vi "Plot PSD.vi"(6 "averaging parameters":T1={"averaging mode"=enum."No averaging", "weighting mode"=enum."Exponential", "number of averages"=10} {"number of averages" min=1}, 7 "restart averaging (F)":bool, 8 "error in (no error)":errorcluster, 9 "dB On (F)":bool, 10 "window":T2=1 items=["Rectangle"=0, "Hanning"=1, "Hamming"=2, "Blackman-Harris"=3, "Exact Blackman"=4, "Blackman"=5, "Flat Top"=6, "4 Term B-Harris "=7, "7 Term B-Harris"=8, "Low Sidelobe"=9, "Blackman Nuttall"=11, "Triangle"=30, "Bartlett-Hanning"=31, "Bohman"=32, "Parzen"=33, "Welch"=34, "Kaiser"=60, "Dolph-Chebyshev"=61, "Gaussian"=62], 11 "data":waveform(dbl)[](array[waveform])) -> (0 "error out":errorcluster, 3 "psd plot":cluster{"magnitude":dbl[], dbl[]}[](array[cluster]))   [LabVIEW 2013]
uses:
  <vilib>/Analysis/4window.llb/windowTd.ctl
  <vilib>/measure/maspectr.llb/FFT Power Spectrum and PSD for N Chan.vi
  <vilib>/measure/NI_MAPro.lvlib
  <vilib>/Analysis/NI_AALPro.lvlib
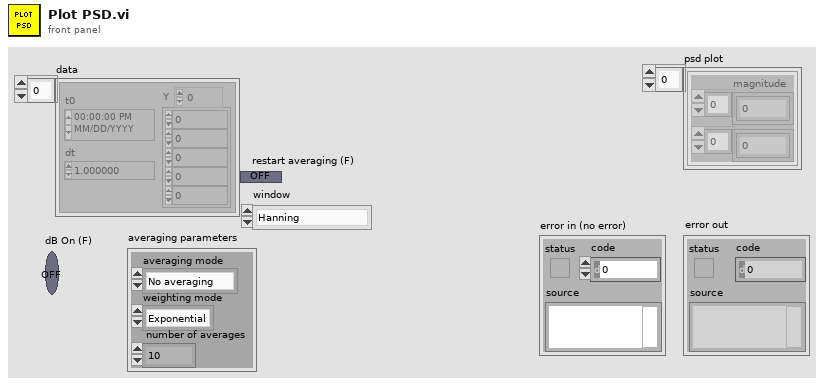
[diagram p1: front panel]
types:
  T1 = cluster{"averaging mode":enum16{"No averaging", "Vector averaging", "RMS averaging", "Peak hold"}, "weighting mode":enum16{"Linear", "Exponential"}, "number of averages":u32}
  T2 = typedef "NI_AALPro.lvlib/windowTd.ctl" = u32
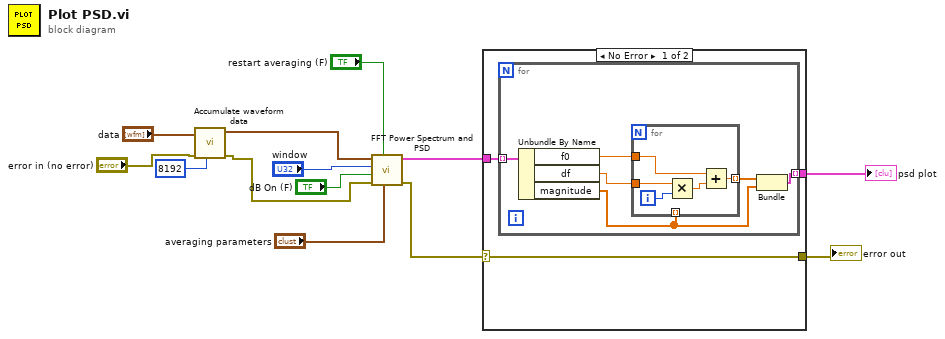
[diagram p0: block diagram]
diagram:
  n1 = call "Accumulate waveform data.vi"("max size"=8192, "error in (no error)"="error in (no error)", "data"="data") -> ("error out"=w2:errorcluster, "data out"=w5:waveform(dbl)[])  [unwired: 7 in]
  n2 = call-poly <vilib>:"FFT Power Spectrum and PSD.vi"("averaging parameters"="averaging parameters", "restart averaging (F)"="restart averaging (F)", "error in (no error)"=w2, "dB On (F)"="dB On (F)", "window"="window", "time signals"=w5) -> ("error out"=w8:errorcluster, "Power Spectrum / PSD"=w13:cluster{"f0":dbl, "df":dbl, "magnitude":dbl[]}[])  [unwired: 2 in, 2 out]
  n3 = case shown="No Error" w8 {
    selector: w8 -> [w14 w28]
    tunnel: w13 -> [w16 _]
    tunnel: [w15 _] -> w1
    tunnel: [w14 w28] -> w7
    frame No Error {
      n4 = for {
        tunnel: w16 -> [w22] mode=indexing
        tunnel: [w18] -> w15 mode=indexing
        n5 = Unbundle By Name(w22) -> ("f0"=w20:dbl, "df"=w21:dbl, "magnitude"=w17:dbl[])
        n6 = for {
          tunnel: w21 -> [w26]
          tunnel: w20 -> [w24]
          tunnel: [w23] -> w19 mode=indexing
          tunnel: w17 -> [_] mode=indexing
          i -> [w27]
          n7 = Multiply(x=w26, y=w27) -> (x*y=w25:dbl)
          n8 = Add(x=w24, y=w25) -> (x+y=w23:dbl)
        }
        n9 = Bundle(w19, "magnitude"=w17) -> (w18:cluster{dbl[], "magnitude":dbl[]})  [unwired: 1 in]
      }
    }
    frame Error {
    }
  }
  "psd plot" <- w1
  "error out" <- w7
